vi "Obtain Leak.vi"(11 "LeakyViewable In":refnum<class "LeakyViewable.lvclass">) -> (1 "Viewable Leak Queue":refnum<queue>, 3 "LeakyViewable Out":refnum<class "LeakyViewable.lvclass">)   [LabVIEW 2017, in "LeakyViewable.lvlib" / "LeakyViewable.lvclass"]
uses:
  LeakyViewable.lvclass
  Leak Location.ctl
  Source/IViewable/IViewable/IViewable.lvclass
  LeakyViewable.lvclass/LeakyViewable.ctl
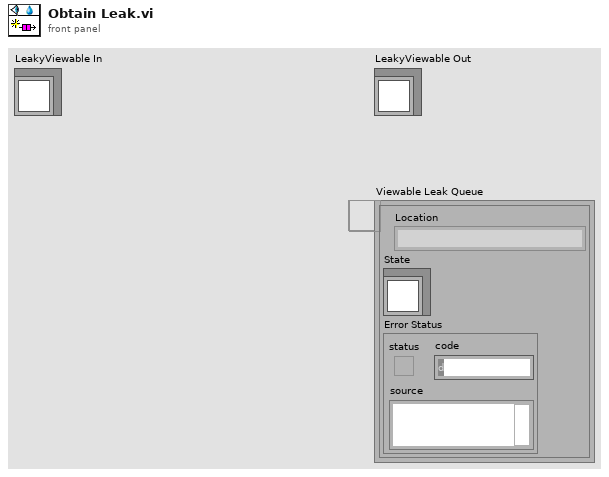
[diagram p1: front panel]
types:
  T1 = typedef "LeakyViewable.lvlib/LeakyViewable.lvclass/Leak Location.ctl" = enum16{"Pre Launch Init", "Entering Actor Core", "Actor Core", "Exiting Actor Core", "Stop Core", "Handle Error"}
  T2 = cluster{"Location":T1, "State":refnum<class "IViewable.lvclass">, "Error Status":errorcluster}
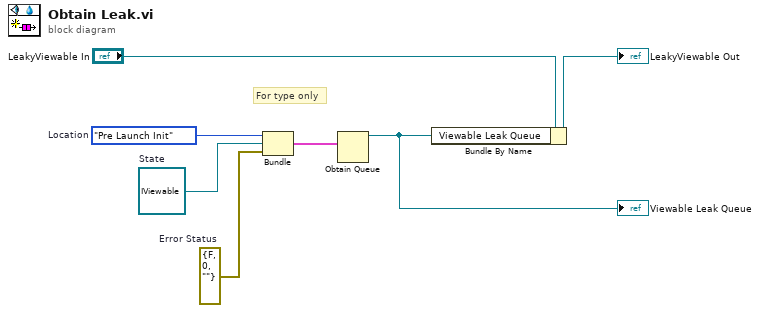
[diagram p0: block diagram]
diagram:
  w3 = errorcluster {"status"=FALSE, "code"=0, "source"=""}  # Error Status
  w5 = Leak_Location."Pre Launch Init"  # Location
  w1 = refnum<class "IViewable.lvclass"> refnum  # State
  # "For type only"
  n1 = Bundle("Location"=w5, "State"=w1, "Error Status"=w3) -> (w4:T2)  [unwired: 1 in]
  n2 = Obtain Queue(element data type=w4) -> (queue out=w2:refnum<queue>)  [unwired: 4 in, 2 out]
  "Viewable Leak Queue" <- w2
  n3 = Bundle By Name(cluster="LeakyViewable In", "Viewable Leak Queue"=w2) -> (→"LeakyViewable Out":refnum<class "LeakyViewable.lvclass">)
